vi "ClimberControl.vi"(10 "Down":bool, 11 "Up":bool) -> ()   [LabVIEW 2012]
uses:
  <vilib>/Rock Robotics/WPI/Relay/WPI_RelayValue.ctl
panel:
  in  "Overite Motor":bool
  in  "Motor Overide":dbl
  in  "Speed":dbl
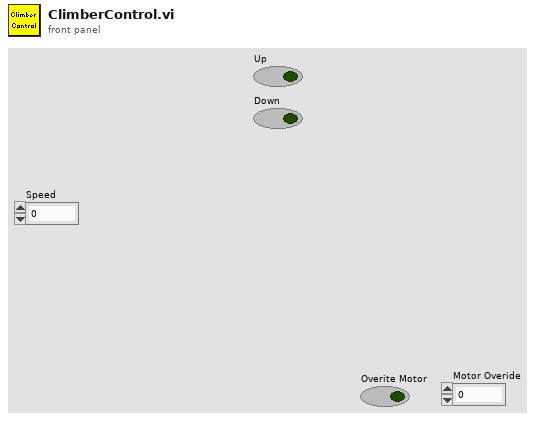
[diagram p1: front panel]
types:
  T1 = typedef "WPI_DigitalInputDevRef.ctl" = cluster{"DevStatus":errorcluster, "DIO Channel":T2, "Digital Module":T3}
  T2 = typedef "FPGA_DIOChannel.ctl" = enum8{"DIO 1", "DIO 2", "DIO 3", "DIO 4", "DIO 5", "DIO 6", "DIO 7", "DIO 8", "DIO 9", "DIO 10", "DIO 11", "DIO 12", "DIO 13", "DIO 14", "Invalid"}
  T3 = typedef "FPGA_TypedefDigitalModule.ctl" = enum16{"Digital Module 1", "Digital Module 2"}
  T4 = typedef "WPI_RelayValue.ctl" = enum16{"Off", "On", "Forward", "Reverse"}
  T5 = typedef "WPI_MotorControlDeviceRef.ctl" = cluster{"DeviceStatus":errorcluster, "Type":enum16{"PWM", "CAN"}, "PWM":cluster{"Digital Module":T3, "PWM Channel":T6, "DeadBand":T7}, "CAN":cluster{"Device Number":u8, "Control Mode":T8, "Semaphore":T9, "Max Vout":dbl}, "Invert":bool, "TransformRef":T10, "InvTransformRef":T10}
  T6 = typedef "FPGA_DIOPWMChannel.ctl" = enum8{"PWM 1", "PWM 2", "PWM 3", "PWM 4", "PWM 5", "PWM 6", "PWM 7", "PWM 8", "PWM 9", "PWM 10", "Invalid"}
  T7 = typedef "WPI_PWMDeadband.ctl" = cluster{"Name":string, "maxPositivePwm":i32, "minPositivePwm":i32, "centerPwm":i32, "maxNegativePwm":i32, "minNegativePwm":i32, "angularRange":u16}
  T8 = typedef "WPI_CANJaguar_ControlMode.ctl" = enum8{"Percent VBus", "Current", "Speed", "Position", "Voltage"}
  T9 = typedef "Semaphore RefNum" = refnum<k1>
  T10 = typedef "WPI_PWMTransform_ConPane.ctl" = refnum<vi>
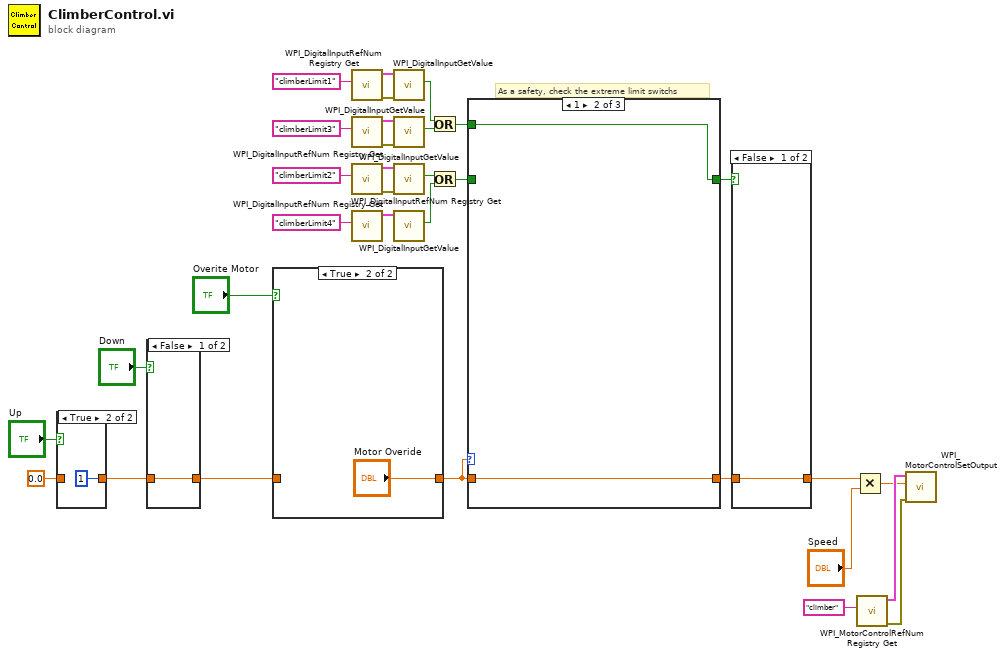
[diagram p0: block diagram]
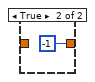
[diagram p2: hidden frame]
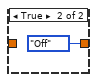
[diagram p5: hidden frame]
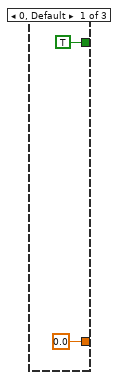
[diagram p6: hidden frame]
diagram:
  # "As a safety, check the extreme limit switchs"
  n1 = case shown="True" "Up" {
    tunnel: [w33 1] -> w3
    tunnel: 0.0 -> [w33 _]
    frame False {
    }
    frame True {
    }
  }
  n2 = case shown="False" "Down" {
    tunnel: w3 -> [w35 _]
    tunnel: [w35 -1] -> w1
    frame False {
    }
    frame True {
    }
  }
  n3 = case shown="True" "Overite Motor" {
    tunnel: w1 -> [w37 _]
    tunnel: [w37 "Motor Overide"] -> w24
    frame False {
    }
    frame True {
    }
  }
  n4 = call <vilib>:"WPI_DigitalInputRefNum Registry Get.vi"("refnum name"="climberLimit1") -> ("error out"=w15:errorcluster, "DigitalInputDevRef"=w16:T1)  [unwired: 9 in]
  n5 = call <vilib>:"WPI_DigitalInputRefNum Registry Get.vi"("refnum name"="climberLimit3") -> ("error out"=w18:errorcluster, "DigitalInputDevRef"=w19:T1)  [unwired: 9 in]
  n6 = call <vilib>:"WPI_DigitalInputRefNum Registry Get.vi"("refnum name"="climberLimit2") -> ("error out"=w9:errorcluster, "DigitalInputDevRef"=w7:T1)  [unwired: 9 in]
  n7 = call <vilib>:"WPI_DigitalInputRefNum Registry Get.vi"("refnum name"="climberLimit4") -> ("DigitalInputDevRef"=w10:T1)  [unwired: 9 in, 1 out]
  n8 = call <vilib>:"WPI_DigitalInputGetValue.vi"("error in (no error)"=w15, "DigitalInputDevRef"=w16) -> ("Value"=w21:bool)  [unwired: 7 in, 2 out]
  n9 = call <vilib>:"WPI_DigitalInputGetValue.vi"("error in (no error)"=w18, "DigitalInputDevRef"=w19) -> ("Value"=w22:bool)  [unwired: 7 in, 2 out]
  n10 = call <vilib>:"WPI_DigitalInputGetValue.vi"("error in (no error)"=w9, "DigitalInputDevRef"=w7) -> ("Value"=w12:bool)  [unwired: 7 in, 2 out]
  n11 = call <vilib>:"WPI_DigitalInputGetValue.vi"("DigitalInputDevRef"=w10) -> ("Value"=w13:bool)  [unwired: 8 in, 2 out]
  n12 = Or(x=w21, y=w22) -> (x .or. y?=w14:bool)
  n13 = Or(x=w12, y=w13) -> (x .or. y?=w6:bool)
  n14 = case shown="1" w24 {
    tunnel: [TRUE ("Value") w41 w43] -> w32
    tunnel: [0.0 w42 w44] -> w31
    tunnel: w24 -> [_ w42 w44]
    tunnel: w14 -> [_ w41 _]
    tunnel: w6 -> [_ _ w43]
    frame 0, Default {
    }
    frame 1 {
    }
    frame -1 {
    }
  }
  n15 = case shown="False" w32 {
    tunnel: [w45 WPI_RelayValue."Off" ("RelayValue")] -> w29
    tunnel: w31 -> [w45 _]
    frame False {
    }
    frame True {
    }
  }
  n16 = Multiply(x=w29, y="Speed") -> (x*y=w25:dbl)
  n17 = call <vilib>:"WPI_MotorControlRefNum Registry Get.vi"("refnum name"="climber") -> ("error out"=w27:errorcluster, "MotorControlDevRef"=w26:T5)  [unwired: 9 in]
  n18 = call <vilib>:"WPI_MotorControlSetOutput.vi"("error in (no error)"=w27, "Output"=w25, "MotorControlDevRef"=w26) -> ()  [unwired: 6 in, 3 out]
